vi "FTW-WebServer-Construct.vi"(5 "Address":string, 11 "error in":errorcluster) -> (4 "FTW-Router Out":refnum<class "FTW-WebServer.lvclass">, 6 "Actual Address":string, 10 "Event Registration Refnum":refnum<event-registration>, 15 "error out":errorcluster)   [LabVIEW 2015, in "FTW-WebServer.lvclass"]
uses:
  FTW-WebServer.lvclass
  Message/Request/FTW-Message-IncomingRequest.lvclass
  Ether/FTW-Ether-EndpointType.ctl
  FTW-WebServer.lvclass/FTW-WebServer.ctl
  Endpoint/FTW-Endpoint.lvclass
  Ether/FTW-Ether.lvclass
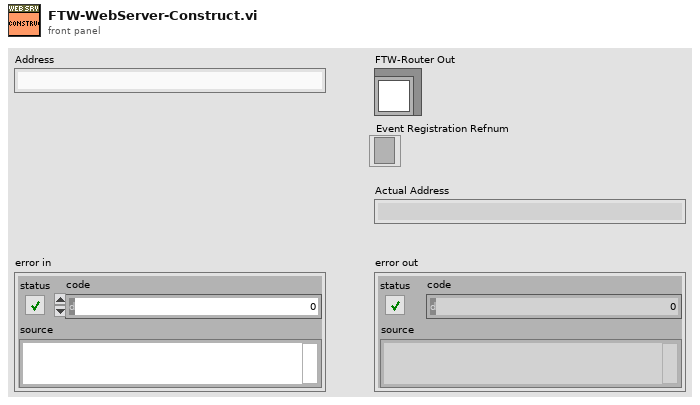
[diagram p1: front panel]
types:
  T1 = typedef "FTW-Ether.lvclass/FTW-Ether-EndpointType.ctl" = enum16{"Server", "Client", "Publisher", "Subscriber"}
  T2 = typedef "FTW-Ether.lvclass/FTW-Ether-MessageTransportScheme.ctl" = enum16{"In process (inproc://)", "TCP (tcp://)"}
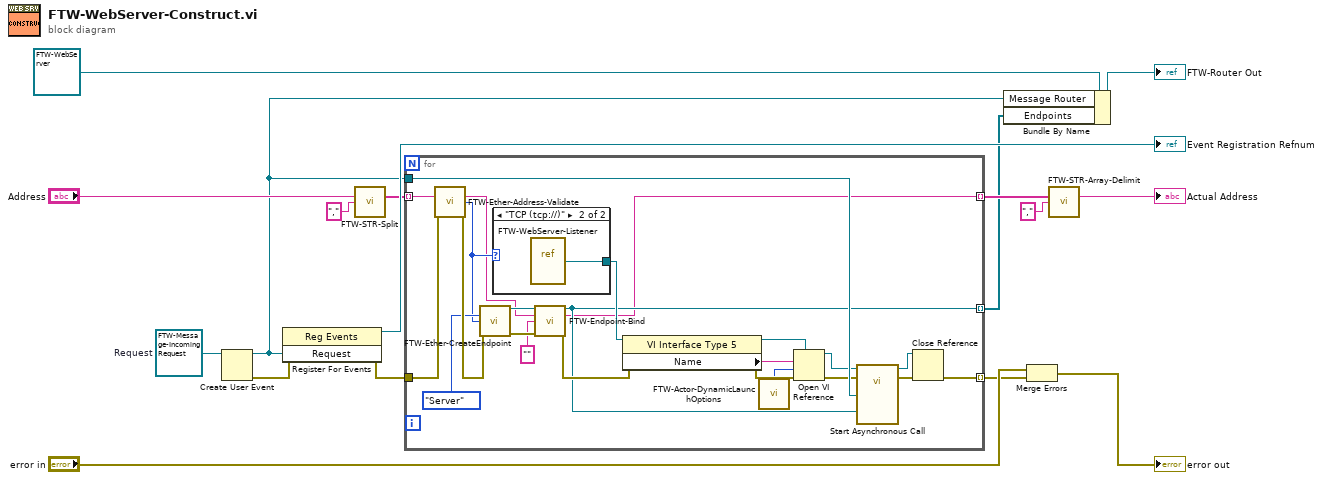
[diagram p0: block diagram]
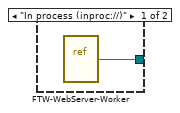
[diagram p2: hidden frame]
diagram:
  w10 = refnum<class "FTW-Message-IncomingRequest.lvclass"> refnum  # Request
  n1 = Create User Event(user event datatype=w10) -> (user event=w8:refnum<user-event>, error out=w6:errorcluster)  [unwired: 1 in]
  n2 = register-events(error in=w6, w8) -> (reference out=→"Event Registration Refnum":refnum<event-registration>, error out=w2:errorcluster)  [unwired: 1 in]
  n3 = call "FTW-STR-Split.vi"("Delimited String"="Address", "Delimiter"=",") -> ("Array of Strings"=w1:string[])  [unwired: 13 in]
  n4 = for {
    tunnel: [w18] -> w9 mode=indexing
    tunnel: w8 -> [w39]
    tunnel: w2 -> [w37]
    tunnel: [w36] -> w7 mode=indexing
    tunnel: w1 -> [w35] mode=indexing
    tunnel: [w21] -> w4 mode=indexing
    n5 = call "FTW-Ether-Address-Validate.vi"("Address"=w35, "error in"=w37) -> ("Sanitized Address"=w19:string, "Message Transport Scheme"=w24:T2, "error out"=w40:errorcluster)  [unwired: 11 in]
    n6 = call "FTW-Ether-CreateEndpoint.vi"("Endpoint Type"=FTW-Ether-EndpointType."Server", "Message Transport Scheme"=w24, "error in"=w40) -> ("FTW Endpoint"=w22:refnum<class "FTW-Endpoint.lvclass">, "error out"=w38:errorcluster)  [unwired: 11 in]
    n7 = case shown="\"TCP (tcp://)\"" w24 {
      tunnel: [w41 w42] -> w33
      frame "In process (inproc://)" {
        n8 = vi-ref "FTW-WebServer-Worker.vi"() -> (w41:refnum<vi>)
      }
      frame "TCP (tcp://)" {
        n9 = vi-ref "FTW-WebServer-Listener.vi"() -> (w42:refnum<vi>)
      }
    }
    n10 = call-dynamic "FTW-Endpoint-Bind.vi"("FTW Endpoint"=w22, "Endpoint Address"=w19, "Requested Identity"="", "error in"=w38) -> ("FTW Endpoint out"=w21:refnum<class "FTW-Endpoint.lvclass">, "Actual Endpoint Address"=w18:string, "error out"=w23:errorcluster)  [unwired: 8 in, 1 out]
    n11 = property class="VI Interface Type 5"(reference=w33, error in=w23) -> (reference out=w29:refnum<vi>, error out=w32:errorcluster, "Name"=w31:string)
    n12 = call "FTW-Actor-DynamicLaunchOptions.vi"() -> ("Open VI Ref Options"=w30:i32)
    n13 = Open VI Reference(type specifier VI Refnum (for type only)=w29, vi path=w31, options=w30, error in (no error)=w32) -> (vi reference=w27:refnum<vi>, error out=w25:errorcluster)  [unwired: 2 in]
    n14 = call-by-ref "Start Asynchronous Call"(reference=w27, error in=w25, "Endpoint"=w21, "Message Handler"=w39) -> (reference out=w26:refnum<vi>, error out=w28:errorcluster)  [unwired: 1 in]
    n15 = Close Reference(reference=w26, error in (no error)=w28) -> (error out=w36:errorcluster)
  }
  n16 = Bundle By Name(cluster=refnum<class "FTW-WebServer.lvclass"> refnum ("LVmsg_Router.lvclass"), "Message Router"=w8, "Endpoints"=w4) -> (→"FTW-Router Out":refnum<class "FTW-WebServer.lvclass">)
  n17 = Merge Errors("error in", w7) -> (→"error out":errorcluster)
  n18 = call "FTW-STR-Array-Delimit.vi"("Array of Strings"=w9, "Delimiter"=",") -> ("Delimited String"=→"Actual Address":string)  [unwired: 13 in]
